vi "Get AI Limit Configuration.vi"(8 "error in (no error)":errorcluster) -> (0 "error out":errorcluster, 3 "AI LIMIT out":T1(array[cluster]))   [LabVIEW 2018]
uses:
  <vilib>/Utility/xml.llb/Read From XML File(string).vi
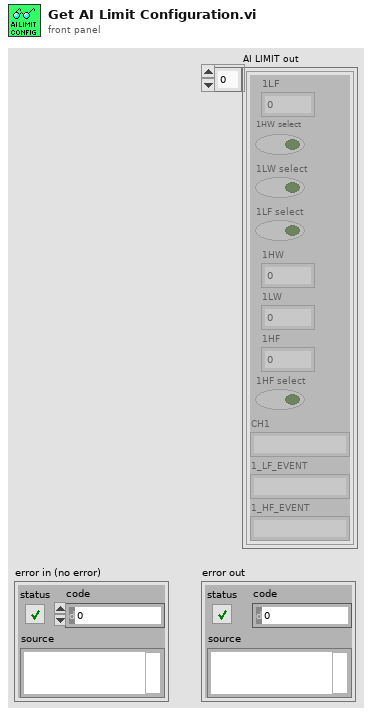
[diagram p1: front panel]
types:
  T1 = cluster{"1LF":dbl, "1HW select":bool, "1LW select":bool, "1LF select":bool, "1HW":dbl, "1LW":dbl, "1HF":dbl, "1HF select":bool, "CH1":string, "1_LF_EVENT":string, "1_HF_EVENT":string}[]
  T2 = typedef "Limit Paths.ctl" = cluster{"Limit 1 Config Path":path, "Limit 2 Config Path ":path, "Limit 3 Config Path ":path, "Limit 4 Config Path ":path, "Limit 5 Config Path ":path, "Limit 6 Config Path ":path, "CallimitPath ":path}
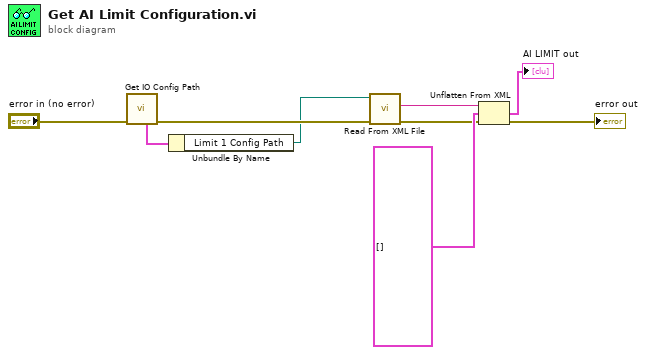
[diagram p0: block diagram]
diagram:
  n1 = call "Get IO Config Path.vi"("error in (no error)"="error in (no error)") -> ("error out"=w9:errorcluster, "Limit Path"=w7:T2)  [unwired: 5 in, 4 out]
  n2 = Unbundle By Name(w7) -> ("Limit 1 Config Path"=w8:path)
  n3 = call-poly <vilib>:"Read From XML File.vi"("error in (no error)"=w9, "XML File Path"=w8) -> ("error out"=w1:errorcluster, "XML Elements"=w2:string)  [unwired: 7 in, 1 out]
  n4 = Unflatten From XML(xml string=w2, type=T1 [] ("Type Specifier"), error in (no error)=w1) -> (value=→"AI LIMIT out":T1, error out=→"error out":errorcluster)
